vi "计算因法兰旋转导致的坐标偏移.vi"(9 "旋转半径":dbl, 10 "机械手当前角度":dbl, 11 "旋转角度":dbl) -> (2 "dtx,dty Out":T1 {"X" format="%#.3f"})   [LabVIEW 2014]
uses:
  Controls/XYPos.ctl
panel:
  in  "H0旋转角度(单位角度)":dbl=-69.635 format="%#_13g"
  # "-0.3\n0.488"
  # "0.43  0.9345"
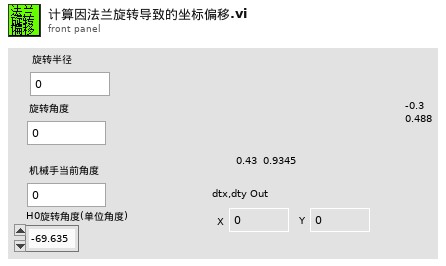
[diagram p1: front panel]
types:
  T1 = typedef "XYPos.ctl" = cluster{"X":dbl, "Y":dbl}
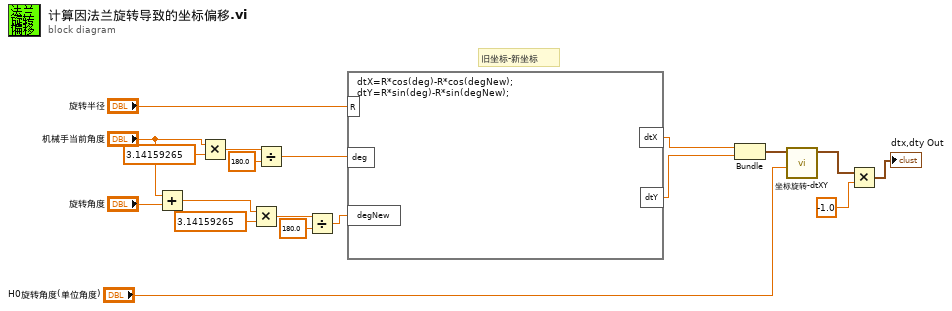
[diagram p0: block diagram]
diagram:
  # "旧坐标-新坐标"
  n1 = Add(x="机械手当前角度", y="旋转角度") -> (x+y=w11:dbl)
  n2 = Multiply(x="机械手当前角度", y=3.14159265) -> (x*y=w18:dbl)
  n3 = Multiply(x=w11, y=3.14159265) -> (x*y=w13:dbl)
  n4 = Divide(x=w18, y=180.0) -> (x/y=w10:dbl)
  n5 = Divide(x=w13, y=180.0) -> (x/y=w9:dbl)
  n6 = formula code="dtX=R*cos(deg)-R*cos(degNew);\ndtY=R*sin(deg)-R*sin(degNew);"("R"="旋转半径", "deg"=w10, "degNew"=w9) -> ("dtX"=w7:dbl, "dtY"=w6:dbl)
  n7 = Bundle("dtX"=w7, "dtY"=w6) -> (w5:cluster{"dtX":dbl, "dtY":dbl})  [unwired: 1 in]
  n8 = call "坐标旋转-dtXY.vi"("旋转角度(单位角度)"="H0旋转角度(单位角度)", "dtx,dty In"=w5) -> ("dtx,dty Out"=w3:T1)  [unwired: 9 in]
  n9 = Multiply(x=w3, y=-1.0) -> (x*y=→"dtx,dty Out":T1)
